vi "Fire LogEngineStateChanged Event_LogEngine.vi"(8 "error in (no error)":errorcluster, 10 "NEW State Data":T1, 11 "LogEngine":refnum<class "LogEngine.lvclass">) -> (0 "error out":errorcluster, 3 "LogEngine out":refnum<class "LogEngine.lvclass">)   [LabVIEW 2017, in "LogEngine.lvclass"]
doc: "Developed by Kevin Thompson\nkevin@thompsonengineering.net\n\nCopyright 2018-2020\nThompson Engineering, LLC"
uses:
  LogEngine.lvclass
  Data Types/TD Logger State Data--cluster.ctl
  Data Types/TD Logger State--enum.ctl
  Data Types/TD LoggerStateChanged EventData--cluster.ctl
  LogEngine.lvclass/LogEngine.ctl
  Accessors/Get Logger State Data.vi
  Accessors/Set Logger State Data.vi
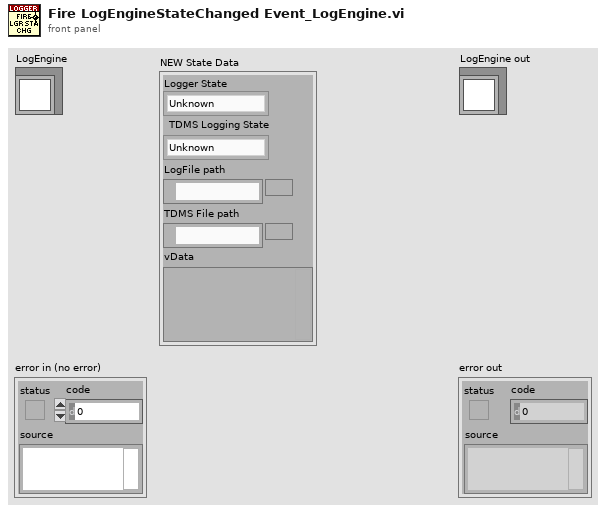
[diagram p1: front panel]
types:
  T1 = typedef "LogEngine.lvclass/TD Logger State Data--cluster.ctl" = cluster{"Logger State":T2, "TDMS Logging State":T2, "LogFile path":path, "TDMS File path":path, "vData":variant}
  T2 = typedef "LogEngine.lvclass/TD Logger State--enum.ctl" = enum16{"Unknown", "Logging", "NotLogging", "Error"}
  T3 = typedef "LogEngine.lvclass/TD LoggerStateChanged EventData--cluster.ctl" = cluster{"Time Stamp":timestamp, "OLD State Data":T1, "NEW State Data":T1}
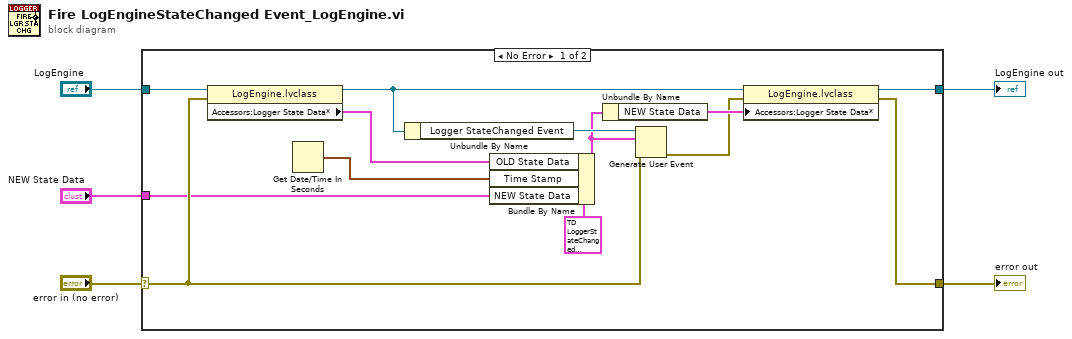
[diagram p0: block diagram]
diagram:
  n1 = case shown="No Error" "error in (no error)" {
    selector: "error in (no error)" -> [w7 w20]
    tunnel: [w9 w20] -> w4
    tunnel: [w13 w19] -> w3
    tunnel: "LogEngine" -> [w16 w19]
    tunnel: "NEW State Data" -> [w6 _]
    frame No Error {
      n2 = property class="LogEngine.lvclass"(reference=w16, error in=w7) -> (reference out=w14:refnum<class "LogEngine.lvclass">, "Accessors:Logger State Data*"=w15:T1)  [unwired: 1 out]
      n3 = Get Date/Time In Seconds() -> (seconds since 1Jan1904=w17:timestamp)
      n4 = Unbundle By Name(w14) -> ("Logger StateChanged Event"=w18:refnum<user-event>)
      n5 = Bundle By Name(cluster=T3 {"Time Stamp"=timestamp(0 s since 1904-01-01), "OLD State Data"={"Logger State"=enum."Unknown", "TDMS Logging State"=enum."Unknown", "LogFile path"=path "", "TDMS File path"=path "", "vData"=variant}, "NEW State Data"={"Logger State"=enum."Unknown", "TDMS Logging State"=enum."Unknown", "LogFile path"=path "", "TDMS File path"=path "", "vData"=variant}} ("DAQStateChanged EventData"), "OLD State Data"=w15, "Time Stamp"=w17, "NEW State Data"=w6) -> (w12:T3)
      n6 = Unbundle By Name(w12) -> ("NEW State Data"=w11:T1)
      n7 = Generate User Event(user event=w18, event data cluster=w12, error in=w7) -> (error out=w10:errorcluster)  [unwired: 1 in, 1 out]
      n8 = property class="LogEngine.lvclass"(reference=w14, error in=w10, "Accessors:Logger State Data*"=w11) -> (reference out=w13:refnum<class "LogEngine.lvclass">, error out=w9:errorcluster)
    }
    frame Error {
    }
  }
  "error out" <- w4
  "LogEngine out" <- w3
